vi "20201007 sensor pick and place test data space.vi"() -> ()   [LabVIEW 2016]
panel:
  out "Standard Dev 3":dbl
  out "RMS 3":dbl
  out "Arithmetic Mean 3":dbl
  out "Standard Dev 2":dbl
  out "RMS 2":dbl
  out "Arithmetic Mean 2":dbl
  out "Standard Dev":dbl
  out "RMS":dbl
  out "Arithmetic Mean":dbl
  out "Histogram 3":dynamicdata(graph) caption="Histogram"
  out "Histogram 2":dynamicdata(graph) caption="Histogram"
  out "Histogram":dynamicdata(graph)
  out "X2":dbl[](array[numeric])
  out "Y2":dbl[](array[numeric])
  out "R2":dbl[](array[numeric])
  out "X pos":dbl format="%#_13g"
  out "Y pos":dbl format="%#_13g"
  out "rotation":dbl format="%#_13g"
  # "Total test times : 25\nThre results are subtracted by the target position already."
  # "Y"
  # "y position"
  # "X position"
  # "rotation"
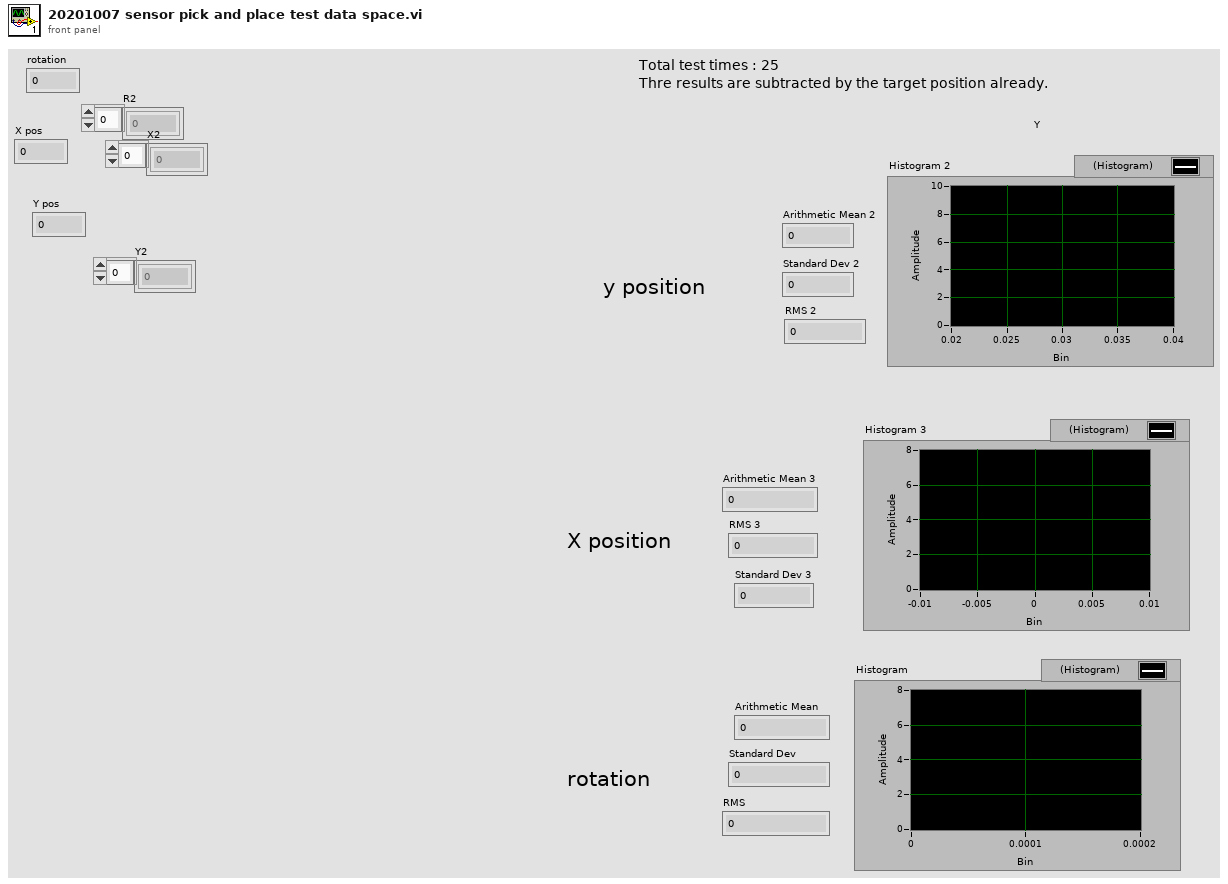
[diagram p1: front panel]
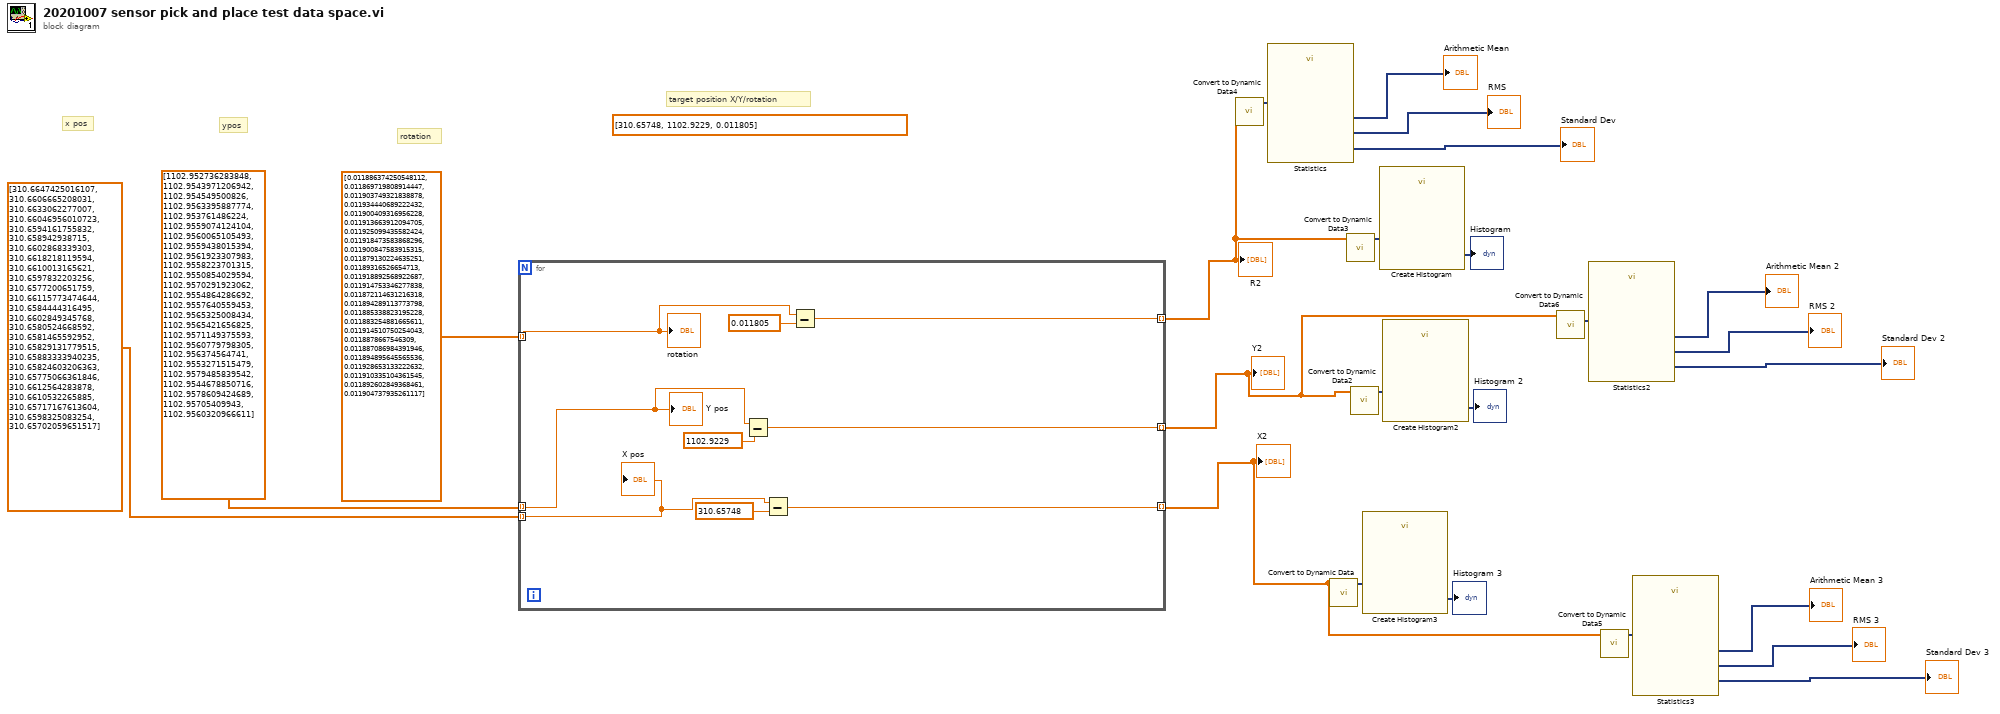
[diagram p0: block diagram]
diagram:
  (unwired) dbl[] [310.65748, 1102.9229, 0.011805]
  # "target position X/Y/rotation"
  # "rotation"
  # "ypos"
  # "x pos"
  n1 = for {
    tunnel: dbl[] [0.011886374250548112, 0.011869719808914447, 0.011903749321838878, 0.011934440689222432, 0.011900409316956228, 0.011913663912094705, 0.011925099435582424, 0.011918473583868296, 0.011900847583915315, 0.011879130224635251, 0.01189316526654713, 0.011918892568922687, 0.011914753346277838, 0.011872114631216318, 0.011894289113773798, 0.011885338823195228, 0.011883254881665611, 0.011914510750254043, 0.0118878667546309, 0.011887086984391946, 0.011894895645565536, 0.011928653133222632, 0.011910335104361545, 0.011892602849368461, 0.011904737935261117] ("Array") -> [w28] mode=indexing
    tunnel: dbl[] [1102.952736283848, 1102.9543971206942, 1102.954549500826, 1102.9563395887774, 1102.953761486224, 1102.9559074124104, 1102.9560065105493, 1102.9559438015394, 1102.9561923307983, 1102.9558223701315, 1102.9550854029594, 1102.9570291923062, 1102.9554864286692, 1102.9557640559453, 1102.9565325008434, 1102.9565421656825, 1102.9571149375593, 1102.9560779798305, 1102.956374564741, 1102.9553271515479, 1102.9579485839542, 1102.9544678850716, 1102.9578609424689, 1102.95705409943, 1102.9560320966611] ("Yposition") -> [w29] mode=indexing
    tunnel: dbl[] [310.6647425016107, 310.6606665208031, 310.6633062277007, 310.66046956010723, 310.6594161755832, 310.658942938715, 310.6602868339303, 310.6618218119594, 310.6610013165621, 310.6597832203256, 310.6577200651759, 310.66115773474644, 310.6584444316495, 310.6602849345768, 310.6580524668592, 310.6581465592952, 310.65829131779515, 310.65883333940235, 310.65824603206363, 310.65775066361846, 310.6612564283878, 310.6610532265885, 310.65717167613604, 310.6598325083254, 310.65702059651517] ("X position") -> [w30] mode=indexing
    tunnel: [w27] -> w15 mode=indexing
    tunnel: [w26] -> w2 mode=indexing
    tunnel: [w25] -> w4 mode=indexing
    n2 = Subtract(x=w29, y=1102.9229) -> (x-y=w26:dbl)
    n3 = Subtract(x=w30, y=310.65748) -> (x-y=w25:dbl)
    n4 = Subtract(x=w28, y=0.011805) -> (x-y=w27:dbl)
    "rotation" <- w28
    "Y pos" <- w29
    "X pos" <- w30
  }
  "R2" <- w15
  "Y2" <- w2
  "X2" <- w4
  n5 = call "Convert to Dynamic Data4"("Array"=w15) -> ("Dynamic Data Type"=w14:dynamicdata)  [unwired: 3 in]
  n6 = call "Statistics"("Signals"=w14) -> ("Standard Dev"=→"Standard Dev":dynamicdata, "RMS"=→"RMS":dynamicdata, "Arithmetic Mean"=→"Arithmetic Mean":dynamicdata)  [unwired: 23 in, 1 out]
  n7 = call "Convert to Dynamic Data"("Array"=w4) -> ("Dynamic Data Type"=w18:dynamicdata)  [unwired: 3 in]
  n8 = call "Convert to Dynamic Data3"("Array"=w15) -> ("Dynamic Data Type"=w16:dynamicdata)  [unwired: 3 in]
  n9 = call "Convert to Dynamic Data2"("Array"=w2) -> ("Dynamic Data Type"=w17:dynamicdata)  [unwired: 3 in]
  n10 = call "Create Histogram3"("Signal"=w18) -> ("Histogram"=→"Histogram 3":dynamicdata)  [unwired: 9 in, 1 out]
  n11 = call "Create Histogram"("Signal"=w16) -> ("Histogram"=→"Histogram":dynamicdata)  [unwired: 9 in, 1 out]
  n12 = call "Create Histogram2"("Signal"=w17) -> ("Histogram"=→"Histogram 2":dynamicdata)  [unwired: 9 in, 1 out]
  n13 = call "Convert to Dynamic Data6"("Array"=w2) -> ("Dynamic Data Type"=w1:dynamicdata)  [unwired: 3 in]
  n14 = call "Statistics2"("Signals"=w1) -> ("Standard Dev"=→"Standard Dev 2":dynamicdata, "RMS"=→"RMS 2":dynamicdata, "Arithmetic Mean"=→"Arithmetic Mean 2":dynamicdata)  [unwired: 23 in, 1 out]
  n15 = call "Convert to Dynamic Data5"("Array"=w4) -> ("Dynamic Data Type"=w3:dynamicdata)  [unwired: 3 in]
  n16 = call "Statistics3"("Signals"=w3) -> ("Standard Dev"=→"Standard Dev 3":dynamicdata, "RMS"=→"RMS 3":dynamicdata, "Arithmetic Mean"=→"Arithmetic Mean 3":dynamicdata)  [unwired: 23 in, 1 out]
